vi "Read clConfigOptions.vi"(8 "error in (no error)":errorcluster, 11 "OutputToFileBasePlugin in":refnum<class "OutputToFileBasePlugin.lvclass">) -> (0 "error out":errorcluster, 2 "clConfigOptions":T1={"TIME_BASE"=1000000, "STN"="Bus_1", "IDCODE"=0, "rdoPolRect"=enum."Rectangular", "rdoFloatInt"=enum."Float", "PHUNIT"=1000000, "rdoFreqDfreq"=enum."Float", "CHNAM"=["VA", "VB", "VC", "V+", "IA", "IB", "IC", "I+"], "chkCfg2Prefix"=TRUE} caption="PMU Configuration Options" {"PHUNIT" max=16777216 step=1 format="%08d"; "IDCODE" format="%02x"; "TIME_BASE" max=16777216 step=1 format="%08d"}, 3 "OutputToFileBasePlugin out":refnum<class "OutputToFileBasePlugin.lvclass">)   [LabVIEW 2017, in "OutputToFilePlugins.lvlib" / "OutputToFileBasePlugin.lvclass"]
uses:
  OutputToFileBasePlugin.lvclass
  Typedefs/PmuCfgOpt.ctl
  OutputToFileBasePlugin.lvclass/OutputToFileBasePlugin.ctl
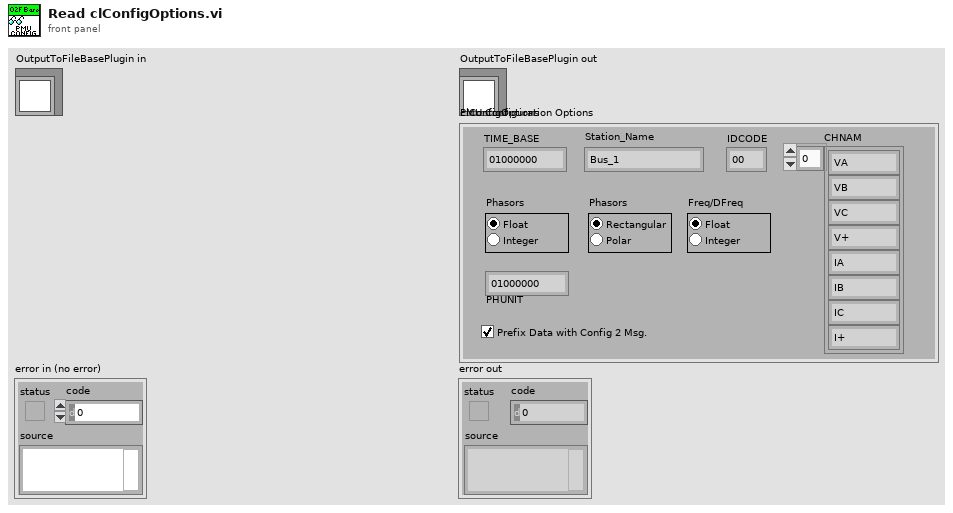
[diagram p1: front panel]
types:
  T1 = typedef "OutputToFilePlugins.lvlib/OutputToFileBasePlugin.lvclass/PmuCfgOpt.ctl" = cluster{"TIME_BASE":u64, "STN":string, "IDCODE":u16, "rdoPolRect":enum32{"Rectangular", "Polar"}, "rdoFloatInt":enum32{"Float", "Integer"}, "PHUNIT":u64, "rdoFreqDfreq":enum32{"Float", "Integer"}, "CHNAM":string[], "chkCfg2Prefix":bool}
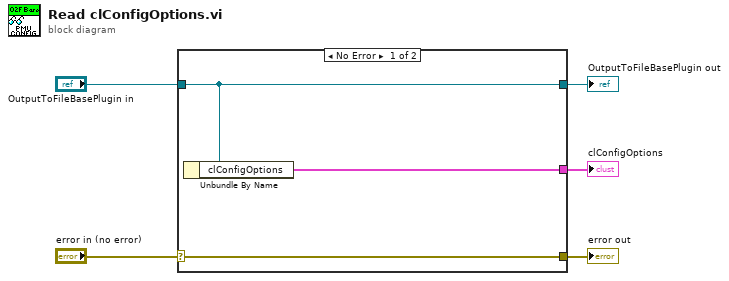
[diagram p0: block diagram]
diagram:
  n1 = case shown="No Error" "error in (no error)" {
    selector: "error in (no error)" -> [w8 w9]
    tunnel: [w8 w9] -> w4
    tunnel: [w7 w10] -> w2
    tunnel: "OutputToFileBasePlugin in" -> [w7 w10]
    tunnel: [w6 _] -> w1
    frame No Error {
      n2 = Unbundle By Name(w7) -> ("clConfigOptions"=w6:T1)
    }
    frame Error {
    }
  }
  "error out" <- w4
  "OutputToFileBasePlugin out" <- w2
  "clConfigOptions" <- w1
